vi "lecture2-SubVIs.vi"(2 "Numeric 2":dbl, 4 "Numeric":dbl) -> (0 "x/y":dbl)   [LabVIEW 2014]
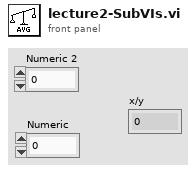
[diagram p1: front panel]
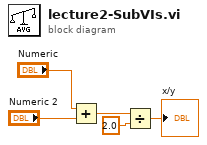
[diagram p0: block diagram]
diagram:
  n1 = Add(x="Numeric", y="Numeric 2") -> (x+y=w3:dbl)
  n2 = Divide(x=w3, y=2.0) -> (x/y=→"x/y":dbl)
